vi "Finish.vi"   [LabVIEW 2019]
doc: "This VI is called just before exiting. It is expected to close I/O refnum, save collected data, etc."
uses:
  <vilib>/Rock Robotics/WPI/Utilities/WPI_GetSetVariantRefNum.vi
  <vilib>/Rock Robotics/WPI/Ultrasonic/WPI_SonarSRF04DigitalRefNum Registry Get.vi
  <vilib>/Rock Robotics/WPI/Ultrasonic/WPI_SonarSRF04DigitalClose.vi
types:
  T1 = typedef "WPI_MotorControlDeviceRef.ctl" = cluster{"DeviceStatus":errorcluster, "Type":T2, "PWM":cluster{"PWM Channel":T3, "DeadBand":T4}, "CAN":cluster{"Device Number":u8, "SetOutput VI Ref":variant, "GetOutput VI Ref":variant, "Enable VI Ref":variant, "Disable VI Ref":variant, "Data":variant}, "Invert":bool, "DIO PWM":cluster{"PWM \"Enable\" Channel":T3, "DIOChannel":T5, "PWM Rate":dbl}}
  T2 = typedef "WPI_MotorControlType.ctl" = enum16{"PWM", "CAN", "DIO PWM"}
  T3 = typedef "FPGA_DIOPWMChannel.ctl" = enum8{"PWM 0", "PWM 1", "PWM 2", "PWM 3", "PWM 4", "PWM 5", "PWM 6", "PWM 7", "PWM 8", "PWM 9", "PWM MXP 0", "PWM MXP 1", "PWM MXP 2", "PWM MXP 3", "PWM MXP 4", "PWM MXP 5", "PWM MXP 6", "PWM MXP 7", "PWM MXP 8", "PWM MXP 9", "Invalid"}
  T4 = typedef "WPI_PWMDeadband.ctl" = cluster{"Name":string, "maxPositivePwm":i32, "minPositivePwm":i32, "centerPwm":i32, "maxNegativePwm":i32, "minNegativePwm":i32, "angularRange":u16}
  T5 = typedef "FPGA_DIOChannel.ctl" = enum8{"DIO 0", "DIO 1", "DIO 2", "DIO 3", "DIO 4", "DIO 5", "DIO 6", "DIO 7", "DIO 8", "DIO 9", "DIO MXP 0", "DIO MXP 1", "DIO MXP 2", "DIO MXP 3", "DIO MXP 4", "DIO MXP 5", "DIO MXP 6", "DIO MXP 7", "DIO MXP 8", "DIO MXP 9", "DIO MXP 10", "DIO MXP 11", "DIO MXP 12", "DIO MXP 13", "DIO MXP 14", "DIO MXP 15", "SPI Port CS1", "SPI Port CS2", "SPI Port CS3", "SPI Port MISO", "SPI Port MOSI", "Invalid"}
  T6 = typedef "WPI_CompressorDevRef.ctl" = cluster{"DevStatus":errorcluster, "Pneumatics Control Module":u8}
  T7 = typedef "WPI_UltrasonicDeviceRef.ctl" = cluster{"DevStatus":errorcluster, "Ping Channel":T5, "Echo Channel":T5, "CntIndex":T8}
  T8 = typedef "FPGA_CounterCtrSystemIndex.ctl" = enum8{"Ctr 0", "Ctr 1", "Ctr 2", "Ctr 3", "Ctr 4", "Ctr 5", "Ctr 6", "Ctr 7", "Invalid"}
  T9 = typedef "WPI_AnalogChannelDevRef.ctl" = cluster{"DevStatus":errorcluster, "Analog Channel":T10}
  T10 = typedef "FPGA_AIChannel.ctl" = enum8{"AI 0", "AI 1", "AI 2", "AI 3", "AI MXP 0", "AI MXP 1", "AI MXP 2", "AI MXP 3", "Invalid"}
  T11 = typedef "WPI_PWMDeviceRef.ctl" = cluster{"DeviceStatus":errorcluster, "PWM Channel":T3}
  T12 = typedef "FPGA_DutyCycleDevRef.ctl" = cluster{"DevStatus":errorcluster, "DutyCycleIndex":T13}
  T13 = typedef "FPGA_DutyCycleIndex.ctl" = enum8{"DutyCycle 0", "DutyCycle 1", "DutyCycle 2", "DutyCycle 3", "DutyCycle 4", "DutyCycle 5", "DutyCycle 6", "DutyCycle 7", "Invalid"}
  T14 = typedef "WPI_SolenoidDevRef.ctl" = cluster{"DevStatus":errorcluster, "Pneumatics Control Module":u8, "Forward Solenoid Channel":T15, "Reverse Solenoid Channel":T15}
  T15 = typedef "WPI_SolenoidChannel.ctl" = enum8{"Solenoid 0", "Solenoid 1", "Solenoid 2", "Solenoid 3", "Solenoid 4", "Solenoid 5", "Solenoid 6", "Solenoid 7", "Invalid"}
  T16 = typedef "WPI_JoystickDevRef.ctl" = cluster{"Device":T17}
  T17 = typedef "WPI_JoystickDeviceEnum.ctl" = enum16{"USB 0", "USB 1", "USB 2", "USB 3", "USB 4", "USB 5"}
  T18 = typedef "WPI_RobotDriveDevRef.ctl" = cluster{"DevStatus":errorcluster, "Motors[]":T1[], "Square Inputs":bool, "Max Output":dbl}
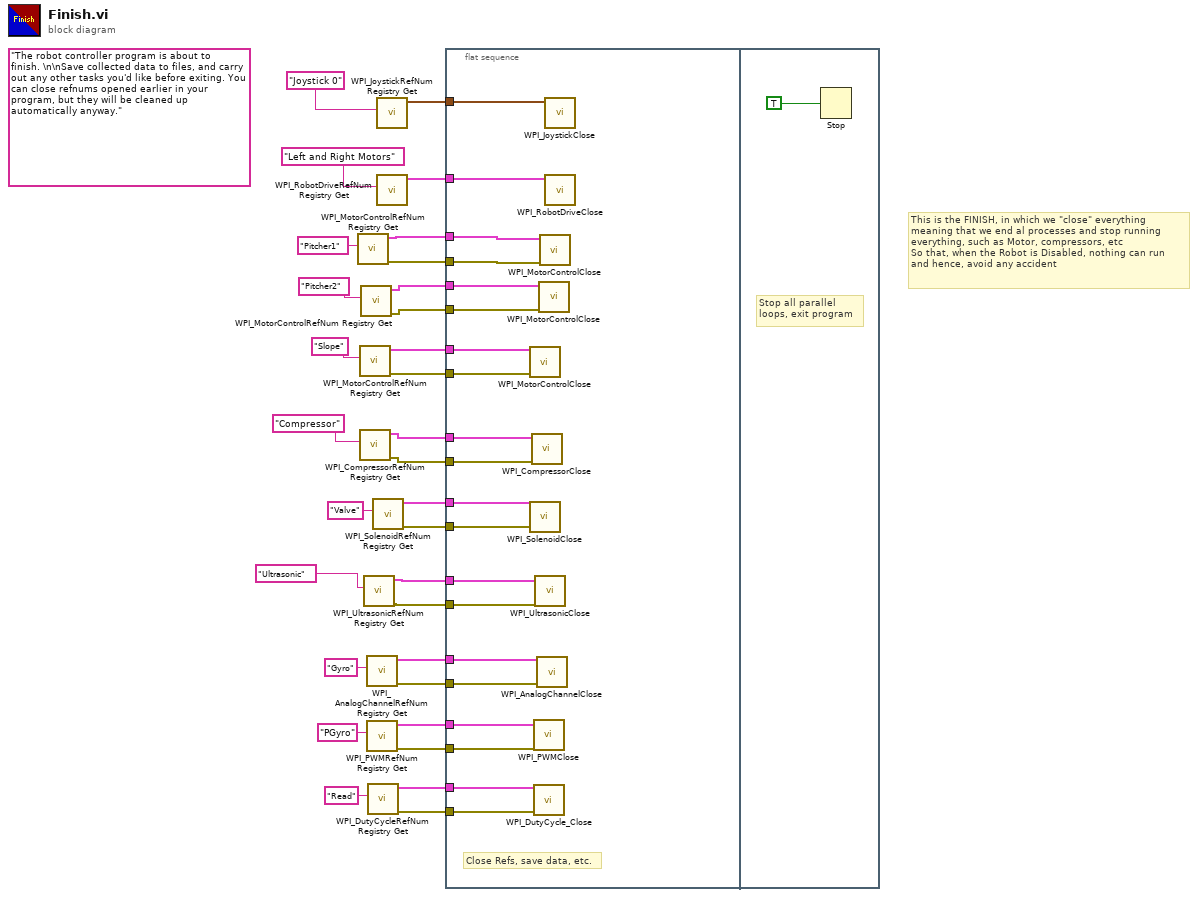
[diagram p0: block diagram]
diagram:
  (unwired) "The robot controller program is about to finish. \n\nSave collected data to files, and carry out any other tasks you'd like before exiting. You can close refnums opened earlier in your program, but they will be cleaned up automatically anyway."
  # "This is the FINISH, in which we \"close\" everything\nmeaning that we end al processes and stop running \neverything, such as Motor, compressors, etc\nSo that, when the Robot is Disabled, nothing can run\nand hence, avoid any accident"
  n1 = call <vilib>:"WPI_MotorControlRefNum Registry Get.vi"("refnum name"="Pitcher1") -> ("error out"=w26:errorcluster, "MotorControlDevRef"=w27:T1)  [unwired: 9 in]
  n2 = call <vilib>:"WPI_MotorControlRefNum Registry Get.vi"("refnum name"="Slope") -> ("error out"=w19:errorcluster, "MotorControlDevRef"=w20:T1)  [unwired: 9 in]
  n3 = call <vilib>:"WPI_CompressorRefNum Registry Get.vi"("refnum name"="Compressor") -> ("error out"=w17:errorcluster, "CompressorDevRef"=w18:T6)  [unwired: 9 in]
  n4 = call <vilib>:"WPI_MotorControlRefNum Registry Get.vi"("refnum name"="Pitcher2") -> ("error out"=w22:errorcluster, "MotorControlDevRef"=w23:T1)  [unwired: 9 in]
  n5 = call-poly <vilib>:"WPI_UltrasonicRefNum Registry Get.vi"("refnum name"="Ultrasonic") -> ("error out"=w11:errorcluster, "SonarSRF04DevRef"=w12:T7)  [unwired: 9 in]
  n6 = call <vilib>:"WPI_AnalogChannelRefNum Registry Get.vi"("refnum name"="Gyro") -> ("error out"=w8:errorcluster, "AIDeviceRef"=w9:T9)  [unwired: 9 in]
  n7 = call <vilib>:"WPI_PWMRefNum Registry Get.vi"("refnum name"="PGyro") -> ("error out"=w5:errorcluster, "PWMDeviceRef"=w6:T11)  [unwired: 9 in]
  n8 = call <vilib>:"WPI_DutyCycleRefNum Registry Get.vi"("refnum name"="Read") -> ("error out"=w2:errorcluster, "DutyCycleDevRef"=w3:T12)  [unwired: 9 in]
  n9 = call <vilib>:"WPI_SolenoidRefNum Registry Get.vi"("refnum name"="Valve") -> ("error out"=w14:errorcluster, "SolenoidDevRef"=w15:T14)  [unwired: 9 in]
  n10 = call <vilib>:"WPI_JoystickRefNum Registry Get.vi"("refnum name"="Joystick 0") -> ("JoystickDevRef"=w28:T16)  [unwired: 1 in, 9 out]
  n11 = call <vilib>:"WPI_RobotDriveRefNum Registry Get.vi"("refnum name"="Left and Right Motors") -> ("RobotDriveDevRef"=w29:T18)  [unwired: 1 in, 9 out]
  n12 = flat-sequence {
    tunnel: w29 -> [w51]
    tunnel: w28 -> [w50]
    tunnel: w27 -> [w49]
    tunnel: w26 -> [w48]
    tunnel: w23 -> [w47]
    tunnel: w22 -> [w46]
    tunnel: w20 -> [w45]
    tunnel: w19 -> [w44]
    tunnel: w18 -> [w43]
    tunnel: w17 -> [w42]
    tunnel: w15 -> [w41]
    tunnel: w14 -> [w40]
    tunnel: w12 -> [w39]
    tunnel: w11 -> [w38]
    tunnel: w9 -> [w37]
    tunnel: w8 -> [w36]
    tunnel: w6 -> [w35]
    tunnel: w5 -> [w34]
    tunnel: w3 -> [w33]
    tunnel: w2 -> [w32]
    frame #0 {
      # "Close Refs, save data, etc."
      n13 = call <vilib>:"WPI_MotorControlClose.vi"("error in"=w44, "MotorControlDevRef"=w45) -> ()  [unwired: 9 in, 1 out]
      n14 = call <vilib>:"WPI_SolenoidClose.vi"("error in (no error)"=w40, "SolenoidDevRef"=w41) -> ()  [unwired: 9 in, 1 out]
      n15 = call <vilib>:"WPI_CompressorClose.vi"("error in (no error)"=w42, "CompressorDevRef"=w43) -> ()  [unwired: 9 in, 1 out]
      n16 = call <vilib>:"WPI_PWMClose.vi"("error in (no error)"=w34, "PWMDeviceRef"=w35) -> ()  [unwired: 9 in, 1 out]
      n17 = call <vilib>:"WPI_DutyCycle_Close.vi"("error in (no error)"=w32, "DutyCycleDevRef"=w33) -> ()  [unwired: 9 in, 1 out]
      n18 = call-poly <vilib>:"WPI_UltrasonicClose.vi"("error in (no error)"=w38, "SonarSRF04DevRef"=w39) -> ()  [unwired: 9 in, 1 out]
      n19 = call <vilib>:"WPI_AnalogChannelClose.vi"("error in (no error)"=w36, "AIDeviceRef"=w37) -> ()  [unwired: 9 in, 1 out]
      n20 = call <vilib>:"WPI_MotorControlClose.vi"("error in"=w46, "MotorControlDevRef"=w47) -> ()  [unwired: 9 in, 1 out]
      n21 = call <vilib>:"WPI_MotorControlClose.vi"("error in"=w48, "MotorControlDevRef"=w49) -> ()  [unwired: 9 in, 1 out]
      n22 = call <vilib>:"WPI_JoystickClose.vi"("JoystickDevRef"=w50) -> ()  [unwired: 11 out]
      n23 = call <vilib>:"WPI_RobotDriveClose.vi"("RobotDriveDevRef"=w51) -> ()  [unwired: 1 in, 10 out]
    }
    frame #1 {
      # "Stop all parallel\nloops, exit program"
      n24 = Stop(stop? (T)=TRUE ("Quit")) -> ()
    }
  }
